vi "test_Open UDP connection using Clear Error node.vi"(8 "error in (no error)":errorcluster, 11 "TestCase in":refnum<class "Instrument Addon Ethernet Protocol Unit Tests.lvclass">) -> (0 "error out":errorcluster, 3 "TestCase out":refnum<class "Instrument Addon Ethernet Protocol Unit Tests.lvclass">)   [LabVIEW 2023, in "Instrument Addon Ethernet Protocol Unit Tests.lvclass"]
uses:
  Instrument Addon Ethernet Protocol Unit Tests.lvclass
  Instrument Addon Ethernet Protocol Unit Tests.lvclass/Instrument Addon Ethernet Protocol Unit Tests.ctl
  <vilib>/addons/_JKI Toolkits/VI Tester/TestCase.llb/TestCase.lvclass
  UDP/UDP.lvclass
  <vilib>/ErrorRing/Error Ring.xnode
  Constants.vi
  <vilib>/Utility/error.llb/Error Cluster From Error Code.vi
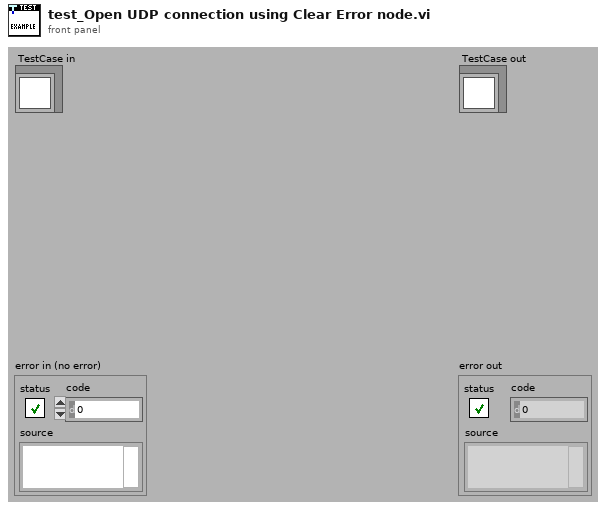
[diagram p1: front panel]
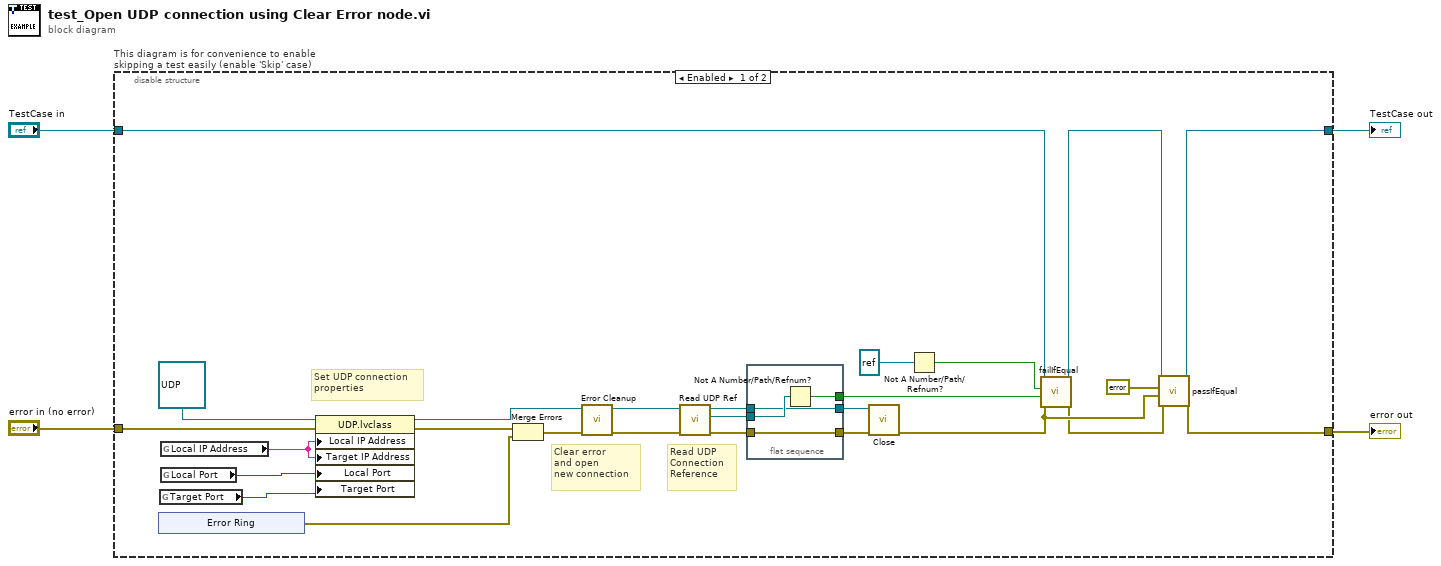
[diagram p0: block diagram]
diagram:
  n1 = disable-structure "This diagram is for convenience to enable skipping a test easily (enable 'Skip' case)" shown="Enabled" {
    disable-tunnel: "TestCase in" -> [w30 w43]
    disable-tunnel: [w13 w41] -> w1
    disable-tunnel: [w11 w42] -> w3
    disable-tunnel: "error in (no error)" -> [w28 w40]
    frame Enabled {
      # "Read UDP\nConnection \nReference"
      # "Clear error \nand open \nnew connection"
      # "Set UDP connection \nproperties"
      n2 = xnode "Error Ring"() -> ("error out"=w25:errorcluster)
      n3 = global read "Constants.vi" "Target Port"() -> (w17:u16)
      n4 = global read "Constants.vi" "Local IP Address"() -> (w19:string)
      n5 = global read "Constants.vi" "Local Port"() -> (w18:u16)
      n6 = property class="UDP.lvclass"(reference=refnum<class "UDP.lvclass"> refnum ("Protocols.lvlib:UDP.lvclass"), error in=w28, "Local IP Address"=w19, "Target IP Address"=w19, "Local Port"=w18, "Target Port"=w17) -> (reference out=w24:refnum<class "UDP.lvclass">, error out=w27:errorcluster)
      n7 = Merge Errors(w27, w25) -> (w26:errorcluster)
      n8 = call-dynamic "Error Cleanup.vi"("error in (no error)"=w26, "UDP in"=w24) -> ("error out"=w23:errorcluster, "UDP out"=w22:refnum<class "UDP.lvclass">)  [unwired: 8 in]
      n9 = call "Read UDP Ref.vi"("error in (no error)"=w23, "UDP in"=w22) -> ("error out"=w10:errorcluster, "UDP Ref"=w7:refnum<k16>, "UDP out"=w8:refnum<class "UDP.lvclass">)  [unwired: 7 in]
      n10 = flat-sequence {
        tunnel: w10 -> [w34]
        tunnel: [w34] -> w9
        tunnel: w8 -> [w31]
        tunnel: w7 -> [w32]
        tunnel: [w33] -> w6
        tunnel: [w31] -> w5
        frame #0 {
          n11 = Not A Number/Path/Refnum?(number/path/refnum=w32) -> (NaN/Path/Refnum?=w33:bool)
        }
      }
      n12 = call-dynamic "Close.vi"("error in (no error)"=w9, "UDP in"=w5) -> ("error out"=w16:errorcluster)  [unwired: 8 in, 1 out]
      n13 = Not A Number/Path/Refnum?(number/path/refnum=refnum<k16> refnum ("UDP Ref")) -> (NaN/Path/Refnum?=w20:bool)
      n14 = call-dynamic "failIfEqual.vi"("error in (no error)"=w16, "y"=w6, "x"=w20, "TestCase in"=w30) -> ("error out"=w15:errorcluster, "TestCase out"=w14:refnum<class "Instrument Addon Ethernet Protocol Unit Tests.lvclass">)  [unwired: 6 in]
      n15 = call-dynamic "passIfEqual.vi"("error in (no error)"=w15, "y"=w16, "x"=errorcluster {"status"=FALSE, "code"=0, "source"=""} ("error constant"), "TestCase in"=w14) -> ("error out"=w11:errorcluster, "TestCase out"=w13:refnum<class "Instrument Addon Ethernet Protocol Unit Tests.lvclass">)  [unwired: 6 in]
    }
    frame Disabled {
      # "skip test result while test is under development"
      n16 = call <vilib>:"skip.vi"("error in (no error)"=w40, "TestCase in"=w43) -> ("error out"=w42:errorcluster, "TestCase out"=w41:refnum<class "Instrument Addon Ethernet Protocol Unit Tests.lvclass">)  [unwired: 8 in]
    }
  }
  "error out" <- w3
  "TestCase out" <- w1
